vi "Diagnose PNS.vi"() -> ()   [LabVIEW 2020, in "PNS.lvlib"]
uses:
  PNS.lvlib
  Visualisierungs Elemente/Button.ctl
  Visualisierungs Elemente/Zahlen-Ausgabefeld.ctl
  ObjektKlassen/Steuerung PNS/Regler.ctl
  Aktionen FGV Istwerte.ctl
  Aktionen FGV Grenzwerte.ctl
  Aktionen FGV Loopkennung.ctl
  Allgemein/allgemeine Sub-VIs.lvlib
  ObjektKlassen/Steuerung PNS/Steuerung PNS.lvclass
panel:
  out "Prop Ausgang %":T1 caption="Prop Ausgang % :" format="%#_5g"
  out "Alarme":string[][](array[string])
  out "Regler":T2
  out "AWC Soll:":T1 caption="AWC Soll" format="%#_5g"
  in  "Beenden":T3
  out "Geräte Adresse:":T1 format="%#_5g"
  out "Geräte Kennung:":T1 format="%#_5g"
  out "Druckluft Störung:":T1 format="%#_5g"
  out "AWC Bitparallel:":T1 format="%#_5g"
  out "AWC Manuell:":T1 format="%#_5g"
  out "AWC Netzwerk:":T1 format="%#_5g"
  out "Auswahl NW/M/BP:":T1 format="%#_5g"
  out "AWC Ist:":T1 format="%#_5g"
  # "Istwerte Probenahmesystem"
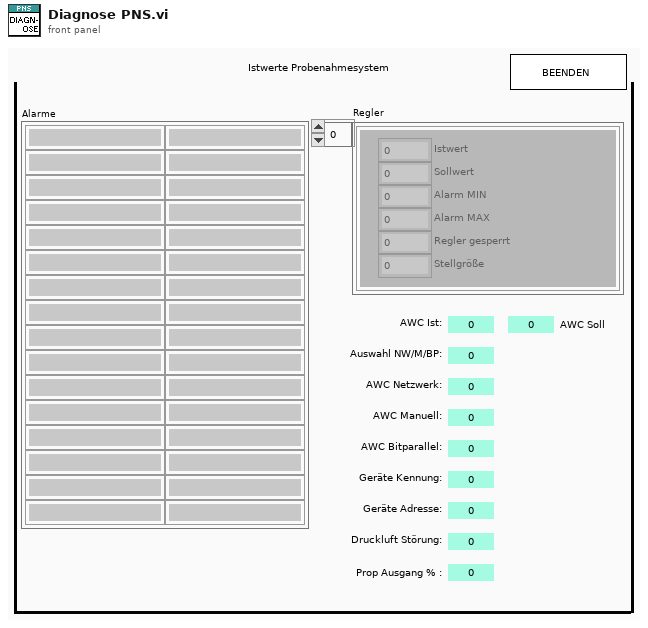
[diagram p1: front panel]
types:
  T1 = typedef "Zahlen-Ausgabefeld.ctl" = sgl
  T2 = typedef "Steuerung PNS.lvclass/Regler.ctl" = cluster{"Istwert":i16, "Sollwert":i16, "Alarm MIN":i16, "Alarm MAX":i16, "Regler sperren":i16, "Analog Ausgang":i16}[]
  T3 = typedef "Button.ctl" = bool
  T4 = typedef "PNS.lvlib/Aktionen FGV Loopkennung.ctl" = enum16{"lesen", "schreiben"}
  T5 = typedef "PNS.lvlib/Aktionen FGV Grenzwerte.ctl" = enum16{"lesen", "Grenzw. schreiben", "Anweisungscode", "IP-Adresse", "laden", "speichern", "Anweisungscode vorgeben"}
  T6 = typedef "PNS.lvlib/Aktionen FGV Istwerte.ctl" = enum16{"lesen", "initialisieren", "schreiben", "Störungen"}
  T7 = typedef "Steuerung PNS.lvclass/Alarme.ctl" = cluster{"Alarm Filter max":u16, "Alarm Filter min":u16, "Alarm Ventilplatte max":u16, "Alarm Ventilplatte min":u16, "Alarm HL1 max":u16, "Alarm HL1 min":u16, "Alarm HL2 max":u16, "Alarm HL2 min":u16, "Alarm HL3 max":u16, "Alarm HL3 min":u16, "Alarm HL4 max":u16, "Alarm HL4 min":u16, "Alarm HL5 max":u16, "Alarm HL5 min":u16, "Alarm HL6 max":u16, "Alarm HL6 min":u16}
  T8 = typedef "Steuerung PNS.lvclass/Anlegengrenzwerte PNS.ctl" = cluster{"Filter:":T9, "Ventilplatte:":T9, "Heizleitung 1:":T9, "Heizleitung 2:":T9, "Heizleitung 3:":T9, "Heizleitung 4:":T9, "Heizleitung 5:":T9, "Heizleitung 6:":T9}
  T9 = typedef "Steuerung PNS.lvclass/Anlagengrenzwerte Parameteranzeige.ctl" = cluster{"Sollwert":T10, "Warn-Min":T10, "Warn-Max":T10, "Abschalt-Min":T10, "Abschalt-Max":T10, "Regler":u16, "AnlagenParameter":string}
  T10 = typedef "Zahlen-Eingabefeld.ctl" = sgl
  T11 = typedef "PNS.lvlib/PNS Geraetekennung.ctl" = cluster{"Loops":string[], "Gerätetype":string, "Loopkennung":u16[], "Seriennummer":string, "Geraetekennung":u16, "SoftWare Version":string, "LP Kennung":u16}
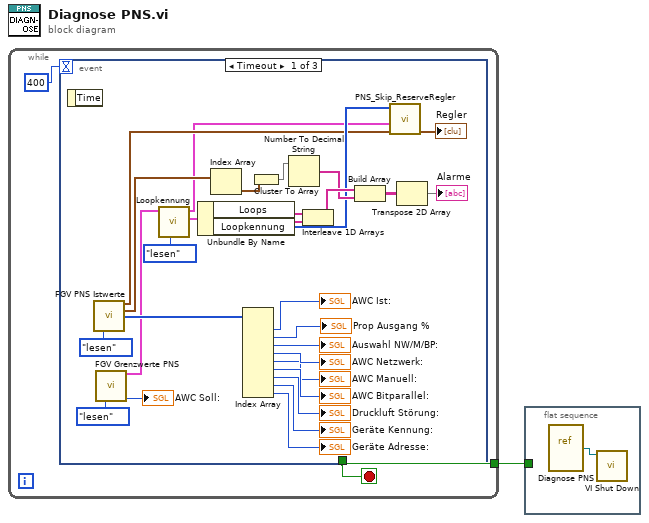
[diagram p0: block diagram]
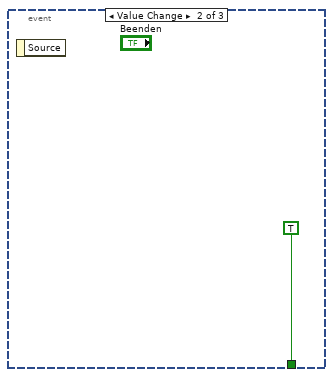
[diagram p2: hidden frame]
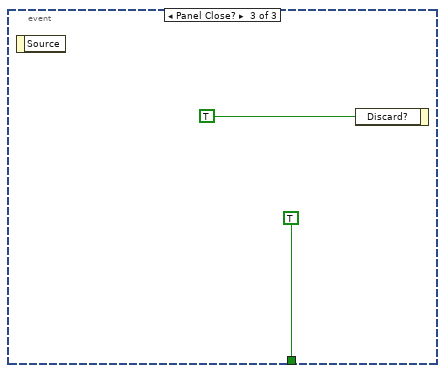
[diagram p3: hidden frame]
diagram:
  n1 = while {
    tunnel: [w2] -> w1
    stop <- w2 stop-if-true
    n2 = event shown="[0] Timeout" {
      selector: _ -> [_ _ _]
      dyn-events: _ -> [_ _ _]
      timeout: 400 -> [_ _ _]
      tunnel: [_ TRUE TRUE] -> w2
      event Timeout {
        n3 = event-data() -> ()  [unwired: 1 in, 1 out]
        n4 = call "FGV PNS Istwerte.vi"("Aktionen"=Aktionen_FGV_Istwerte."lesen") -> ("Regler"=w7:T2, "Alarme"=w15:T7[], "UsrVal"=w10:u16[])  [unwired: 11 in, 1 out]
        n5 = call "FGV Grenzwerte PNS.vi"("Aktionen FGV Grenzwerte"=Aktionen_FGV_Grenzwerte."lesen") -> ("Grenzwerte PNS 2"=w9:T8, "Anweisungscode"=→"AWC Soll:":u16)  [unwired: 12 in, 1 out]
        n6 = call "Loopkennung.vi"("Aktion"=Aktionen_FGV_Loopkennung."lesen", "Grenzwerte PNS 2"=w9) -> ("LoopGeraetekennung"=w12:T11, "Grenzwerte PNS"=w6:T8)  [unwired: 8 in]
        n7 = Unbundle By Name(w12) -> ("Loops"=w11:string[], "Loopkennung"=w8:u16[])
        n8 = Index Array(array=w15) -> (element=w19:T7)  [unwired: 1 in]
        n9 = Index Array(array=w10) -> (element #1=→"AWC Ist:":u16, element #2=→"Prop Ausgang %":u16, element #3=→"Auswahl NW/M/BP:":u16, element #4=→"AWC Netzwerk:":u16, element #5=→"AWC Manuell:":u16, element #6=→"AWC Bitparallel:":u16, element #7=→"Druckluft Störung:":u16, element #8=→"Geräte Kennung:":u16, element #9=→"Geräte Adresse:":u16)  [unwired: 9 in]
        n10 = Cluster To Array(cluster=w19) -> (array=w13:u16[])
        n11 = Number To Decimal String(number=w13) -> (decimal integer string=w16:string[])  [unwired: 1 in]
        n12 = Interleave 1D Arrays(w11, w11) -> (w17:string[])
        n13 = Build Array(w17, w16) -> (w18:string[][])
        n14 = call "PNS_Skip_ReserveRegler.vi"("Regler in"=w7, "Grenzwerte PNS"=w6, "Loopkennung"=w8) -> ("Regler out"=→"Regler":T2)  [unwired: 8 in]
        n15 = Transpose 2D Array(2D array=w18) -> (transposed array=→"Alarme":string[][])
      }
      event Value Change {
        n16 = event-data() -> ()  [unwired: 1 in, 1 out]
      }
      event Panel Close? {
        n17 = event-data() -> ()  [unwired: 1 in, 1 out]
        n18 = event-data("Discard?"=TRUE ("Verwerfen?")) -> ()  [unwired: 1 in, 1 out]
      }
    }
  }
  n19 = flat-sequence {
    tunnel: w1 -> [_]
    frame #0 {
      n20 = vi-ref "Diagnose PNS.vi"() -> (w35:refnum<vi>)
      n21 = call "VI Shut Down.vi"("VI Referenz"=w35) -> ()  [unwired: 11 in]
    }
  }
